vi "Mask Write Register.vi"(4 "OR mask":u16, 6 "AND mask":u16=65535, 8 "error in (no error)":errorcluster, 10 "address":u16, 11 "device data model in":refnum<class "ICPCON ET Data Model.lvclass">) -> (0 "error out":errorcluster, 3 "device data model out":refnum<class "ICPCON ET Data Model.lvclass">)   [LabVIEW 2021, in "ICPCON ET Data Model.lvclass"]
doc: "Writes the masked value of a single register using an <b>AND mask</b> and an <b>OR mask</b> using the equation below:\nResult=(Current Value AND AndMask) OR (OrMask AND !AndMask)"
uses:
  ICPCON ET Data Model.lvclass
  ICPCON ET Data Model.lvclass/ICPCON ET Data Model.ctl
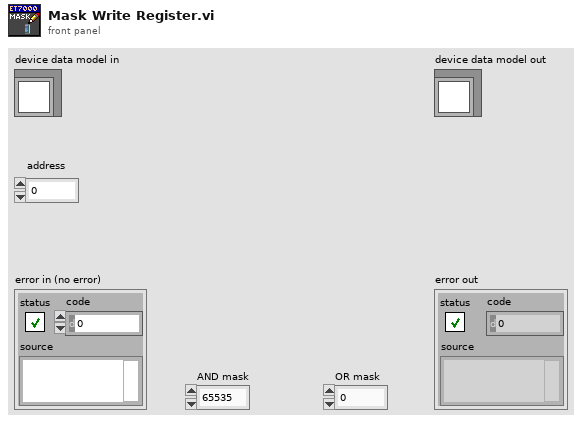
[diagram p1: front panel]
types:
  T1 = typedef "ICPCON ET Data Model.lvclass/Data Model.ctl" = cluster{"UTC":u64, "DI":bool[], "DO":bool[], "IR":u16[], "HR":u16[], "ES":u8}
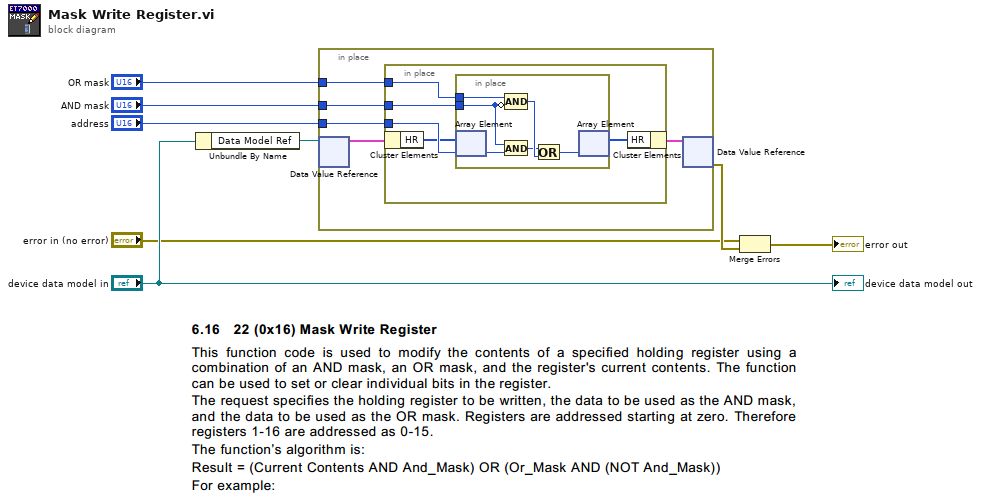
[diagram p0: block diagram]
diagram:
  n1 = Unbundle By Name("device data model in") -> ("Data Model Ref"=w3:refnum<data-value>)
  n2 = in-place {
    in-place-border: "address" -> [w13]
    in-place-border: "AND mask" -> [w12]
    in-place-border: "OR mask" -> [w11]
    n3 = in-place-dvr #1(w3) -> (w9:T1)  [unwired: 1 out]
    n4 = in-place {
      in-place-border: w13 -> [w18]
      in-place-border: w12 -> [w17]
      in-place-border: w11 -> [w16]
      n5 = in-place-cluster #2(w9) -> ("HR"=w15:u16[])
      n6 = in-place {
        in-place-border: w17 -> [w19]
        in-place-border: w16 -> [w21]
        n7 = in-place-array #3(w15, w18) -> (w20:u16)
        n8 = And(x=w19, y=w20) -> (x .and. y?=w23:u16)
        n9 = Compound Arithmetic op=AND(w21, invert w19) -> (w24:u16)
        n10 = Or(x=w23, y=w24) -> (x .or. y?=w22:u16)
        n11 = in-place-array #3(w22) -> (w14:u16[])  [unwired: 1 out]
      }
      n12 = in-place-cluster #2("HR"=w14) -> (w10:T1)
    }
    n13 = in-place-dvr #1(w10) -> (w2:errorcluster)  [unwired: 1 out]
  }
  n14 = Merge Errors("error in (no error)", w2) -> (→"error out":errorcluster)
  "device data model out" <- "device data model in"
